vi "TDMS Async Close.vi"(8 "error in (no error)":errorcluster, 11 "tdms file":refnum<k34>) -> ()   [LabVIEW 2023]
panel:
  out "error out":errorcluster
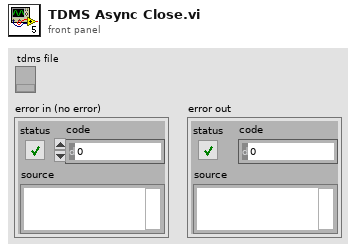
[diagram p1: front panel]
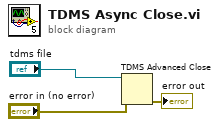
[diagram p0: block diagram]
diagram:
  n1 = TDMS Advanced Close(8:"error in (no error)", 11:"tdms file") -> (0:→"error out":errorcluster)  [unwired: 2 in, 1 out]
